vi "Write Status Display.vi"(8 "error in (no error)":errorcluster, 10 "Status Display":refnum<vi>, 11 "Measurement UI in":refnum<class "Measurement UI.lvclass">) -> (0 "error out":errorcluster, 3 "Measurement UI out":refnum<class "Measurement UI.lvclass">)   [LabVIEW 2015, in "Measurement UI.lvlib" / "Measurement UI.lvclass"]
uses:
  Measurement UI.lvclass
  Measurement UI.lvclass/Measurement UI.ctl
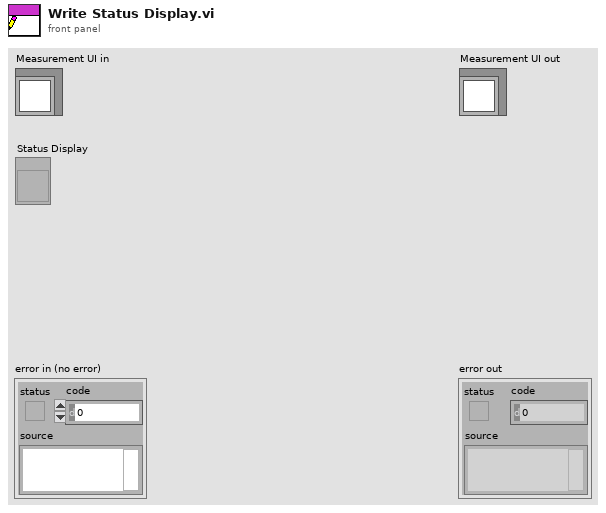
[diagram p1: front panel]
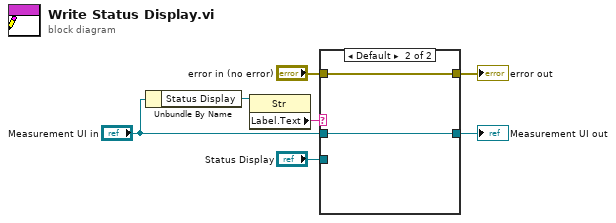
[diagram p0: block diagram]
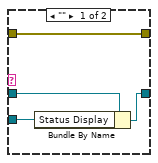
[diagram p2: hidden frame]
diagram:
  n1 = Unbundle By Name("Measurement UI in") -> ("Status Display"=w2:refnum<vi>)
  n2 = property class="Str"(reference=w2) -> ("Label.Text"=w1:string)  [unwired: 1 in, 2 out]
  n3 = case shown="Default" w1 {
    tunnel: [w8 w12] -> w7
    tunnel: [w10 w13] -> w6
    tunnel: "Measurement UI in" -> [w11 w13]
    tunnel: "Status Display" -> [w9 _]
    tunnel: "error in (no error)" -> [w8 w12]
    frame "" {
      n4 = Bundle By Name(cluster=w11, "Status Display"=w9) -> (w10:refnum<class "Measurement UI.lvclass">)
    }
    frame Default {
    }
  }
  "error out" <- w7
  "Measurement UI out" <- w6
